vi "Translator.vi"(0 "Input":variant, 11 "error in (no error)":errorcluster) -> (4 "Output":variant, 15 "error out":errorcluster)   [LabVIEW 2014, in "Arduino Math.lvlib"]
doc: "An example of how to create the Translator to convert the LabVIEW VIs to Arduino C code."
uses:
  <vilib>/Aledyne-TSXperts/Arduino Compatible Compiler for LabVIEW/addons/Arduino Math/Arduino Math.lvlib
panel:
  out "Outputs":string[](array[string])
  out "Inputs":string[](array[string])
  out "Output Datatypes":string[](array[string])
  out "Input Datatypes":string[](array[string])
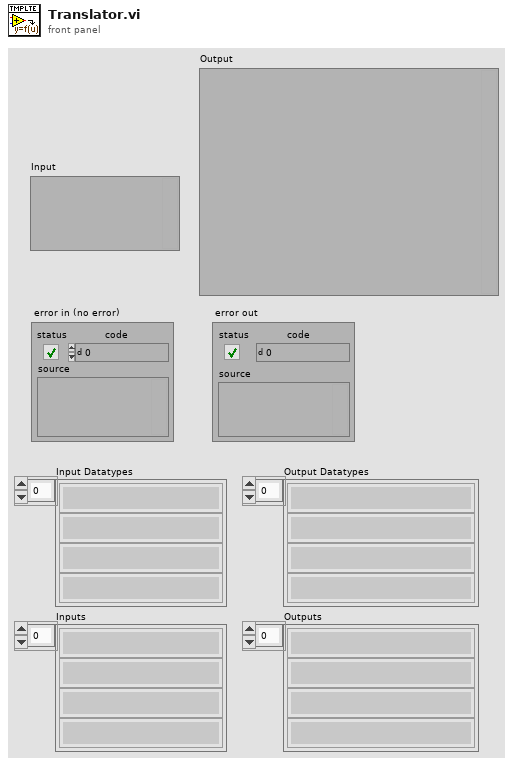
[diagram p1: front panel]
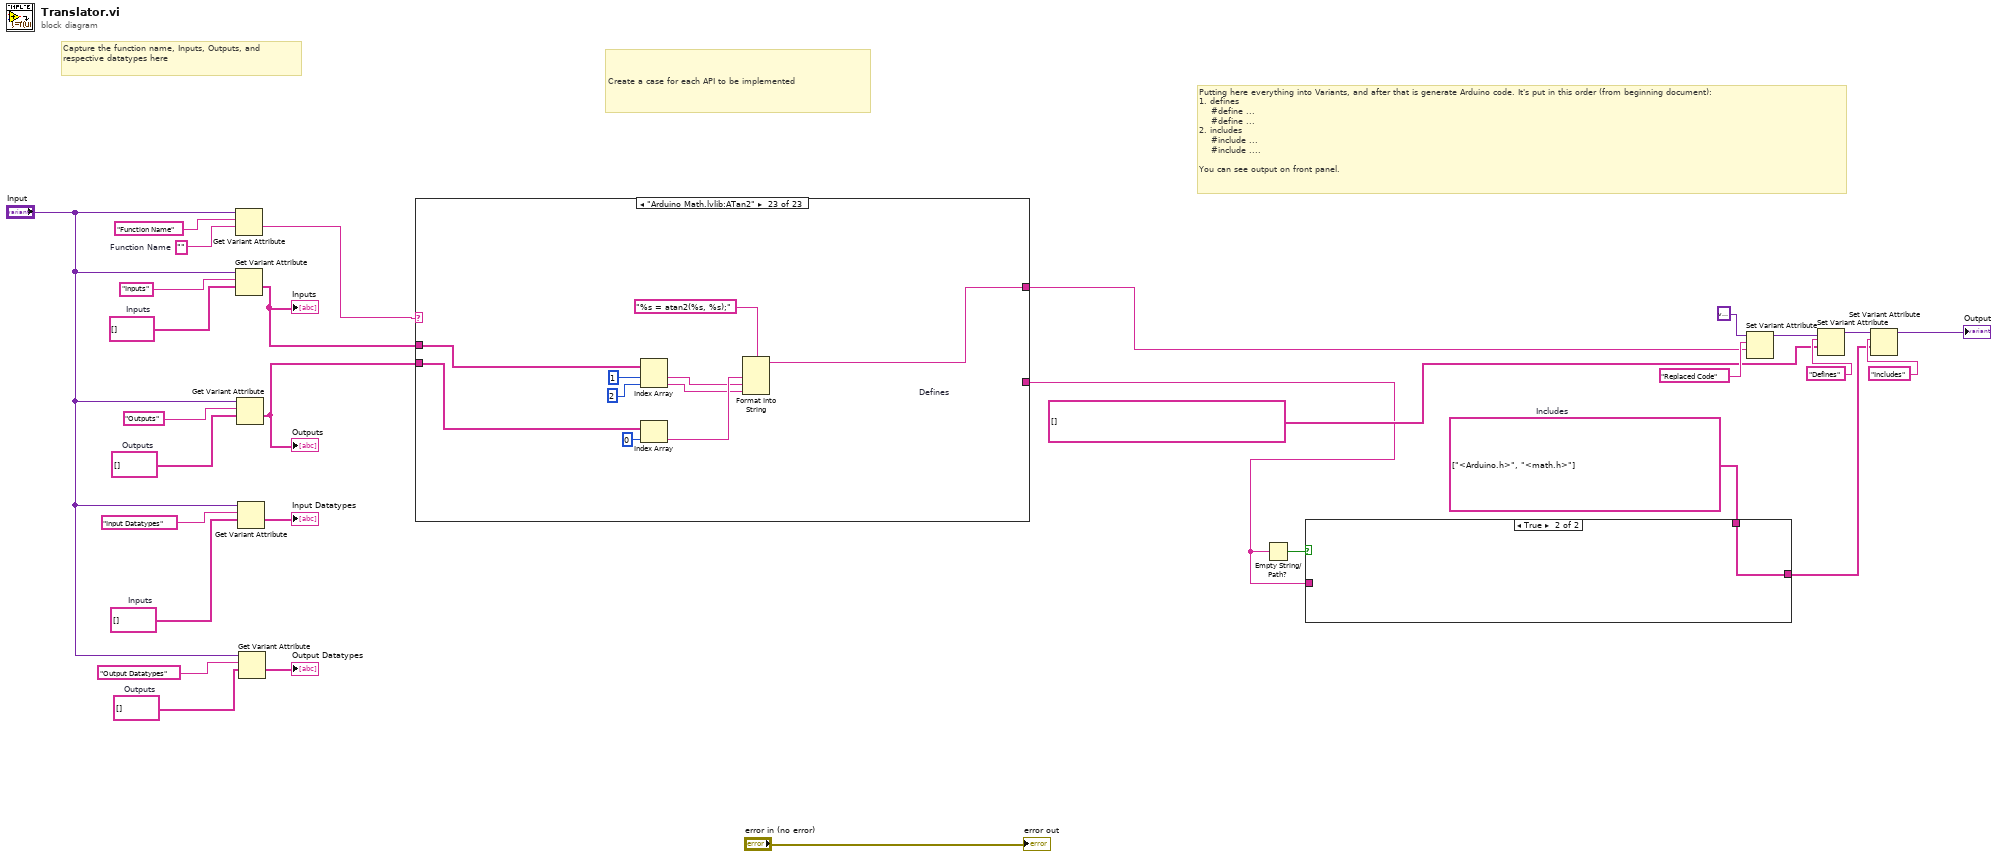
[diagram p0: block diagram]
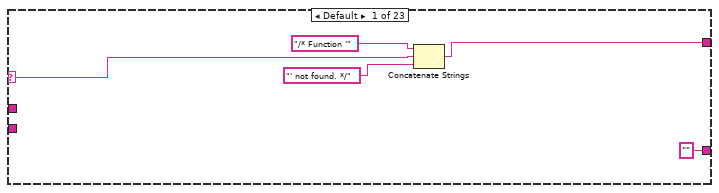
[diagram p2: hidden frame]
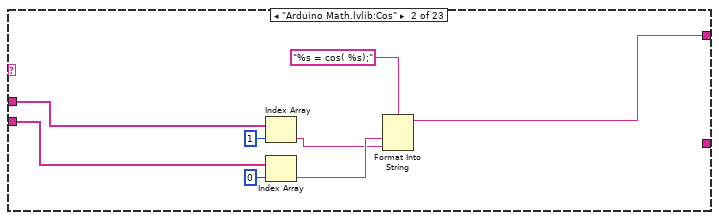
[diagram p3: hidden frame]
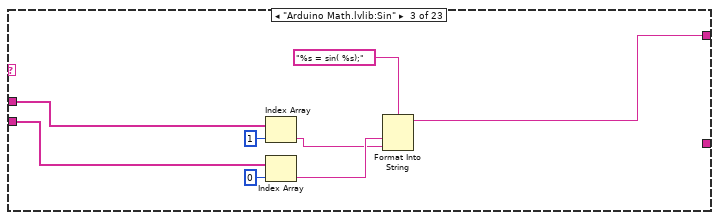
[diagram p4: hidden frame]
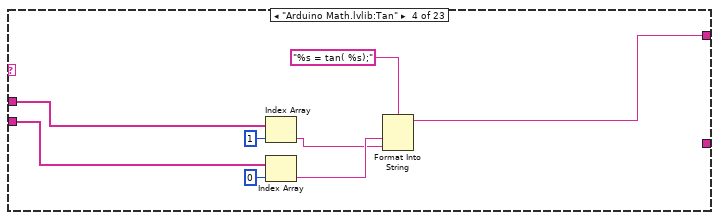
[diagram p5: hidden frame]
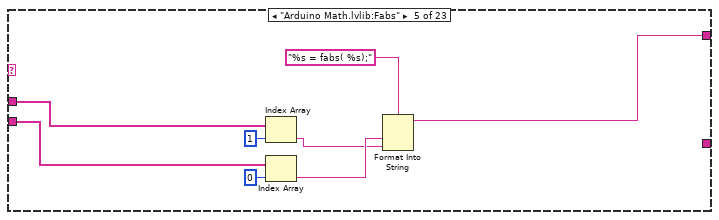
[diagram p6: hidden frame]
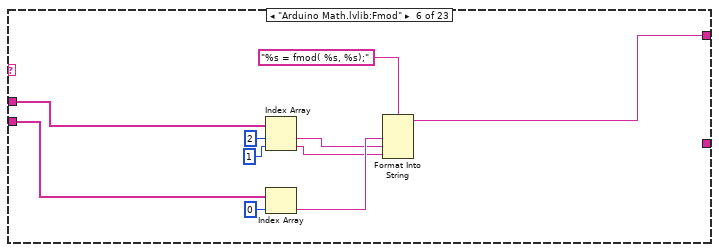
[diagram p7: hidden frame]
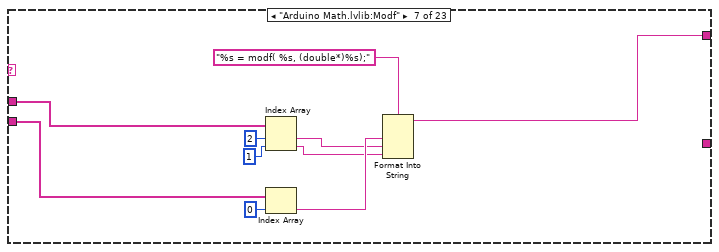
[diagram p8: hidden frame]
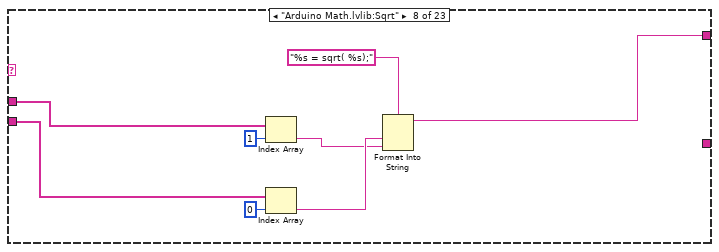
[diagram p9: hidden frame]
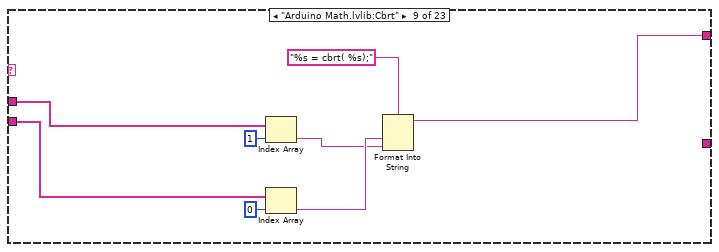
[diagram p10: hidden frame]
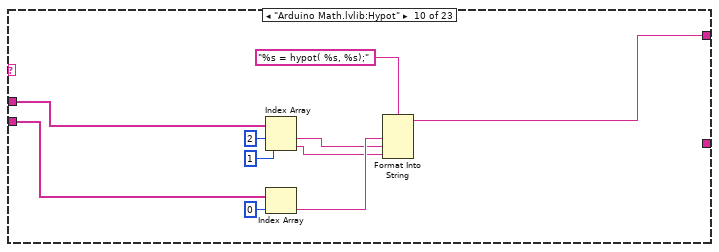
[diagram p11: hidden frame]
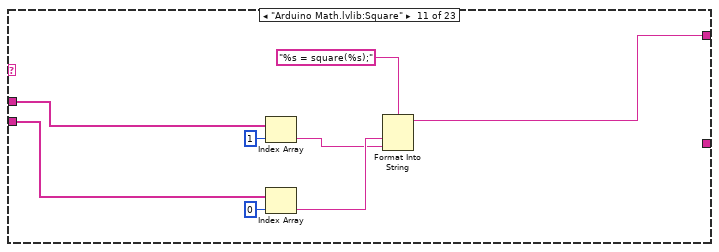
[diagram p12: hidden frame]
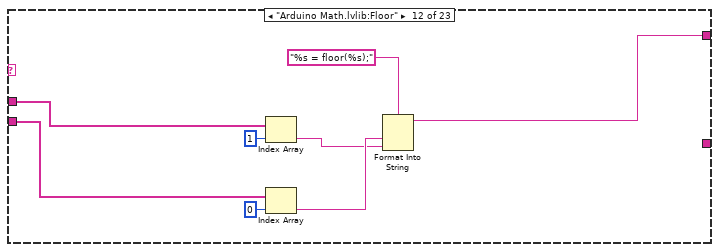
[diagram p13: hidden frame]
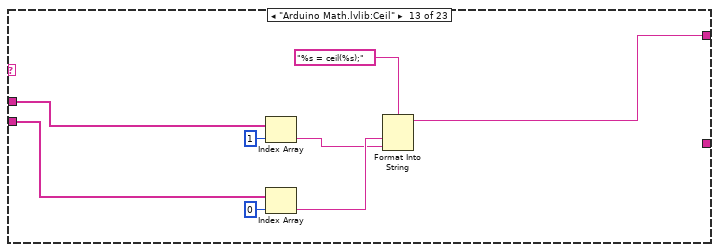
[diagram p14: hidden frame]
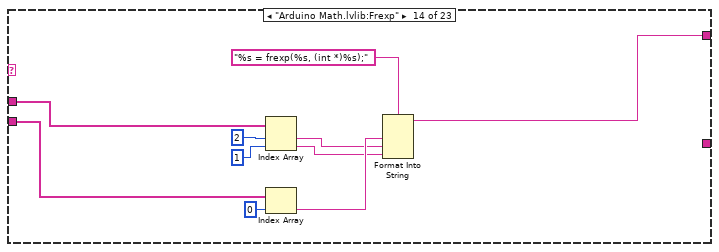
[diagram p15: hidden frame]
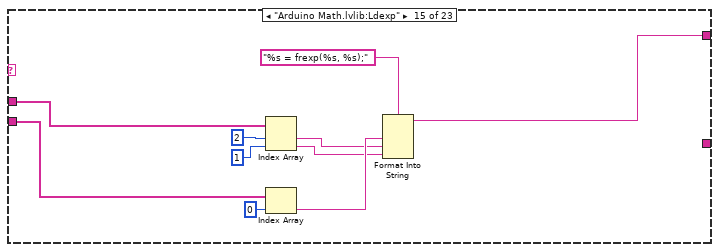
[diagram p16: hidden frame]
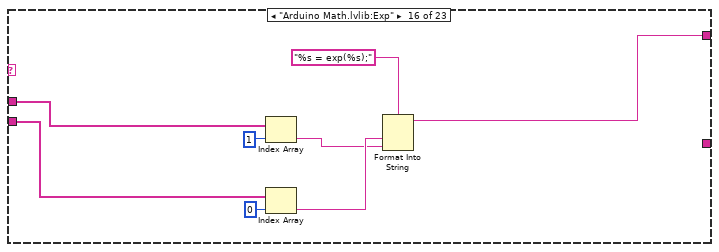
[diagram p17: hidden frame]
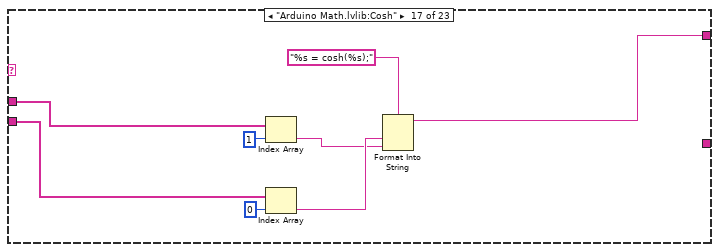
[diagram p18: hidden frame]
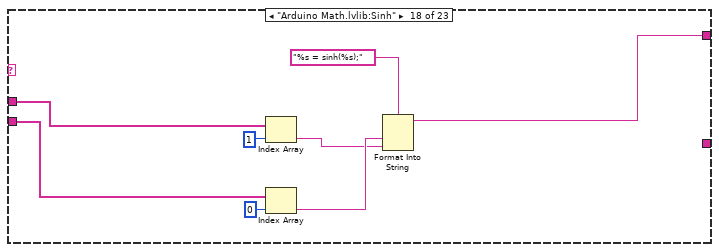
[diagram p19: hidden frame]
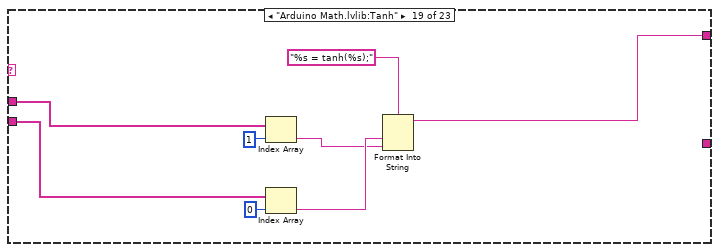
[diagram p20: hidden frame]
diagram:
  w8 = string[] []  # Defines
  w19 = string[] []  # Outputs
  w20 = string[] []  # Inputs
  w6 = string[] ["<Arduino.h>", "<math.h>"]  # Includes
  w26 = string[] []  # Outputs
  w27 = string[] []  # Inputs
  w28 = ""  # Function Name
  # "Capture the function name, Inputs, Outputs, and respective datatypes here"
  # "Putting here everything into Variants, and after that is generate Arduino code. It's put in this order (from beginning document):\n1. defines\n    #define ...\n    #define ...\n2. includes\n    #include ...\n    #include ....\n\nYou can see output on front panel."
  # "Create a case for each API to be implemented"
  n1 = Get Variant Attribute(Variant="Input", name="Function Name", default value (empty Variant)=w28) -> (value=w5:string)  [unwired: 1 in, 3 out]
  n2 = Get Variant Attribute(Variant="Input", name="Inputs", default value (empty Variant)=w27) -> (value=w4:string[])  [unwired: 1 in, 3 out]
  "Inputs" <- w4
  n3 = Get Variant Attribute(Variant="Input", name="Outputs", default value (empty Variant)=w26) -> (value=w3:string[])  [unwired: 1 in, 3 out]
  "Outputs" <- w3
  n4 = Get Variant Attribute(Variant="Input", name="Input Datatypes", default value (empty Variant)=w20) -> (value=→"Input Datatypes":string[])  [unwired: 1 in, 3 out]
  n5 = Get Variant Attribute(Variant="Input", name="Output Datatypes", default value (empty Variant)=w19) -> (value=→"Output Datatypes":string[])  [unwired: 1 in, 3 out]
  n6 = case shown="\"Arduino Math.lvlib:ATan2\"" w5 {
    selector: w5 -> [w35 _ _ _ _ _ _ _ _ _ _ _ _ _ _ _ _ _ _ _ _ _ _]
    tunnel: w4 -> [_ w43 w51 w59 w67 w77 w87 w95 w103 w113 w121 w129 w137 w147 w157 w165 w173 w181 w189 w197 w205 w213 w223]
    tunnel: w3 -> [_ w41 w49 w57 w65 w75 w85 w93 w101 w111 w119 w127 w135 w145 w155 w163 w171 w179 w187 w195 w203 w211 w221]
    tunnel: ["" _ _ _ _ _ _ _ _ _ _ _ _ _ _ _ _ _ _ _ _ _ _] -> w2
    tunnel: [w32 w36 w44 w52 w60 w70 w80 w88 w96 w106 w114 w122 w130 w140 w150 w158 w166 w174 w182 w190 w198 w206 w216] -> w1
    frame Default {
      n7 = Concatenate Strings("/* Function '", w35, "' not found. */") -> (w32:string)
    }
    frame "Arduino Math.lvlib:Cos" {
      n8 = Index Array(array=w43, index=1) -> (element=w38:string)
      n9 = Index Array(array=w41, index=0) -> (element=w39:string)
      n10 = Format Into String(format string="%s = cos( %s);", w39, w38) -> (resulting string=w36:string)  [unwired: 2 in, 1 out]
    }
    frame "Arduino Math.lvlib:Sin" {
      n11 = Index Array(array=w51, index=1) -> (element=w46:string)
      n12 = Index Array(array=w49, index=0) -> (element=w47:string)
      n13 = Format Into String(format string="%s = sin( %s);", w47, w46) -> (resulting string=w44:string)  [unwired: 2 in, 1 out]
    }
    frame "Arduino Math.lvlib:Tan" {
      n14 = Index Array(array=w59, index=1) -> (element=w54:string)
      n15 = Index Array(array=w57, index=0) -> (element=w55:string)
      n16 = Format Into String(format string="%s = tan( %s);", w55, w54) -> (resulting string=w52:string)  [unwired: 2 in, 1 out]
    }
    frame "Arduino Math.lvlib:Fabs" {
      n17 = Index Array(array=w67, index=1) -> (element=w62:string)
      n18 = Index Array(array=w65, index=0) -> (element=w63:string)
      n19 = Format Into String(format string="%s = fabs( %s);", w63, w62) -> (resulting string=w60:string)  [unwired: 2 in, 1 out]
    }
    frame "Arduino Math.lvlib:Fmod" {
      n20 = Index Array(array=w77, index #1=2 ("index"), index #2=1 ("index")) -> (element #1=w72:string, element #2=w68:string)
      n21 = Index Array(array=w75, index=0) -> (element=w73:string)
      n22 = Format Into String(format string="%s = fmod( %s, %s);", w73, w72, w68) -> (resulting string=w70:string)  [unwired: 2 in, 1 out]
    }
    frame "Arduino Math.lvlib:Modf" {
      n23 = Index Array(array=w87, index #1=2 ("index"), index #2=1 ("index")) -> (element #1=w82:string, element #2=w78:string)
      n24 = Index Array(array=w85, index=0) -> (element=w83:string)
      n25 = Format Into String(format string="%s = modf( %s, (double*)%s);", w83, w82, w78) -> (resulting string=w80:string)  [unwired: 2 in, 1 out]
    }
    frame "Arduino Math.lvlib:Sqrt" {
      n26 = Index Array(array=w95, index=1) -> (element=w90:string)
      n27 = Index Array(array=w93, index=0) -> (element=w91:string)
      n28 = Format Into String(format string="%s = sqrt( %s);", w91, w90) -> (resulting string=w88:string)  [unwired: 2 in, 1 out]
    }
    frame "Arduino Math.lvlib:Cbrt" {
      n29 = Index Array(array=w103, index=1) -> (element=w98:string)
      n30 = Index Array(array=w101, index=0) -> (element=w99:string)
      n31 = Format Into String(format string="%s = cbrt( %s);", w99, w98) -> (resulting string=w96:string)  [unwired: 2 in, 1 out]
    }
    frame "Arduino Math.lvlib:Hypot" {
      n32 = Index Array(array=w113, index #1=2 ("index"), index #2=1 ("index")) -> (element #1=w108:string, element #2=w104:string)
      n33 = Index Array(array=w111, index=0) -> (element=w109:string)
      n34 = Format Into String(format string="%s = hypot( %s, %s);", w109, w108, w104) -> (resulting string=w106:string)  [unwired: 2 in, 1 out]
    }
    frame "Arduino Math.lvlib:Square" {
      n35 = Index Array(array=w121, index=1) -> (element=w116:string)
      n36 = Index Array(array=w119, index=0) -> (element=w117:string)
      n37 = Format Into String(format string="%s = square(%s);", w117, w116) -> (resulting string=w114:string)  [unwired: 2 in, 1 out]
    }
    frame "Arduino Math.lvlib:Floor" {
      n38 = Index Array(array=w129, index=1) -> (element=w124:string)
      n39 = Index Array(array=w127, index=0) -> (element=w125:string)
      n40 = Format Into String(format string="%s = floor(%s);", w125, w124) -> (resulting string=w122:string)  [unwired: 2 in, 1 out]
    }
    frame "Arduino Math.lvlib:Ceil" {
      n41 = Index Array(array=w137, index=1) -> (element=w132:string)
      n42 = Index Array(array=w135, index=0) -> (element=w133:string)
      n43 = Format Into String(format string="%s = ceil(%s);", w133, w132) -> (resulting string=w130:string)  [unwired: 2 in, 1 out]
    }
    frame "Arduino Math.lvlib:Frexp" {
      n44 = Index Array(array=w147, index #1=2 ("index"), index #2=1 ("index")) -> (element #1=w142:string, element #2=w138:string)
      n45 = Index Array(array=w145, index=0) -> (element=w143:string)
      n46 = Format Into String(format string="%s = frexp(%s, (int *)%s);", w143, w142, w138) -> (resulting string=w140:string)  [unwired: 2 in, 1 out]
    }
    frame "Arduino Math.lvlib:Ldexp" {
      n47 = Index Array(array=w157, index #1=2 ("index"), index #2=1 ("index")) -> (element #1=w152:string, element #2=w148:string)
      n48 = Index Array(array=w155, index=0) -> (element=w153:string)
      n49 = Format Into String(format string="%s = frexp(%s, %s);", w153, w152, w148) -> (resulting string=w150:string)  [unwired: 2 in, 1 out]
    }
    frame "Arduino Math.lvlib:Exp" {
      n50 = Index Array(array=w165, index=1) -> (element=w160:string)
      n51 = Index Array(array=w163, index=0) -> (element=w161:string)
      n52 = Format Into String(format string="%s = exp(%s);", w161, w160) -> (resulting string=w158:string)  [unwired: 2 in, 1 out]
    }
    frame "Arduino Math.lvlib:Cosh" {
      n53 = Index Array(array=w173, index=1) -> (element=w168:string)
      n54 = Index Array(array=w171, index=0) -> (element=w169:string)
      n55 = Format Into String(format string="%s = cosh(%s);", w169, w168) -> (resulting string=w166:string)  [unwired: 2 in, 1 out]
    }
    frame "Arduino Math.lvlib:Sinh" {
      n56 = Index Array(array=w181, index=1) -> (element=w176:string)
      n57 = Index Array(array=w179, index=0) -> (element=w177:string)
      n58 = Format Into String(format string="%s = sinh(%s);", w177, w176) -> (resulting string=w174:string)  [unwired: 2 in, 1 out]
    }
    frame "Arduino Math.lvlib:Tanh" {
      n59 = Index Array(array=w189, index=1) -> (element=w184:string)
      n60 = Index Array(array=w187, index=0) -> (element=w185:string)
      n61 = Format Into String(format string="%s = tanh(%s);", w185, w184) -> (resulting string=w182:string)  [unwired: 2 in, 1 out]
    }
    frame "Arduino Math.lvlib:Acos" {
      n62 = Index Array(array=w197, index=1) -> (element=w192:string)
      n63 = Index Array(array=w195, index=0) -> (element=w193:string)
      n64 = Format Into String(format string="%s = acos(%s);", w193, w192) -> (resulting string=w190:string)  [unwired: 2 in, 1 out]
    }
    frame "Arduino Math.lvlib:Asin" {
      n65 = Index Array(array=w205, index=1) -> (element=w200:string)
      n66 = Index Array(array=w203, index=0) -> (element=w201:string)
      n67 = Format Into String(format string="%s = asin(%s);", w201, w200) -> (resulting string=w198:string)  [unwired: 2 in, 1 out]
    }
    frame "Arduino Math.lvlib:Atan" {
      n68 = Index Array(array=w213, index=1) -> (element=w208:string)
      n69 = Index Array(array=w211, index=0) -> (element=w209:string)
      n70 = Format Into String(format string="%s = atan(%s);", w209, w208) -> (resulting string=w206:string)  [unwired: 2 in, 1 out]
    }
    frame "Arduino Math.lvlib:ATan2" {
      n71 = Index Array(array=w223, index #1=1 ("index"), index #2=2 ("index")) -> (element #1=w218:string, element #2=w214:string)
      n72 = Index Array(array=w221, index=0) -> (element=w219:string)
      n73 = Format Into String(format string="%s = atan2(%s, %s);", w219, w218, w214) -> (resulting string=w216:string)  [unwired: 2 in, 1 out]
    }
  }
  n74 = Empty String/Path?(string/path=w2) -> (empty?=w9:bool)
  n75 = case shown="True" w9 {
    tunnel: w2 -> [w232 _]
    tunnel: [w225 w233] -> w7
    tunnel: w6 -> [w224 w233]
    frame False {
      n76 = Build Array(w232) -> (w226:string[])
      n77 = Concatenate Strings("<empty.h>" ("string"), "\r\n", w226, "\r\n") -> (w227:string)
      n78 = Build Array(w227) -> (w231:string[])
      n79 = Build Array (concatenate)(w224, w231) -> (w225:string[])
    }
    frame True {
    }
  }
  n80 = Set Variant Attribute(Variant=variant ("variant"), name="Replaced Code", value=w1) -> (Variant out=w13:variant)  [unwired: 1 in, 2 out]
  n81 = Set Variant Attribute(Variant=w13, name="Defines", value=w8) -> (Variant out=w12:variant)  [unwired: 1 in, 2 out]
  n82 = Set Variant Attribute(Variant=w12, name="Includes", value=w7) -> (Variant out=→"Output":variant)  [unwired: 1 in, 2 out]
  "error out" <- "error in (no error)"
